vi "test1.vi"() -> ()   [LabVIEW 2020]
uses:
  <vilib>/DAQmx/write.llb/DAQmx Write (Digital Wfm 1Chan NSamp).vi
  <vilib>/DAQmx/create/channels.llb/DAQmx Create Channel (DO-Digital Output).vi
  <vilib>/Waveform/DWDTOps.llb/DWDT Digital to Boolean Array.vi
  <vilib>/DAQmx/configure/timing.llb/DAQmx Timing (Sample Clock).vi
  <vilib>/Waveform/DWDTOps.llb/DWDT Uncompress Digital.vi
  <vilib>/DAQmx/miscellaneous.llb/DAQmx Fill In Error Info.vi
  <resource>/objmgr/daqmx.rc
panel:
  out "number of samples written per channel":u32
  out "SampClk.Rate":dbl
  in  "stop":bool
  in  "Generate Stimuli":bool=TRUE
  in  "Sol Stim Parameters":cluster{"Fs":dbl, "Samples":dbl}
  in  "LED Stim Parameters":cluster{"Fs":dbl, "Samples":dbl}
  in  "Sol Duty Cycle (%)":dbl=10.0
  in  "Sol Freq":dbl=1.0
  in  "Sol Dur (s)":dbl=1.0
  in  "LED Duty Cycle (%)":dbl=10.0
  in  "LED Freq":dbl=10.0
  in  "LED Dur (s)":dbl=2.0
  out "Stimulus Order":digitalwaveform[](graph)=[{"t0"=timestamp(0 s since 1904-01-01), "dt"=5e-05, "Y"={"transitions"=[], "data"=array18000000x1[18000000 elements]}}, {"t0"=timestamp(0 s since 1904-01-01), "dt"=5e-05, "Y"={"transitions"=[], "data"=array18000000x1[18000000 elements]}}, {"t0"=timestamp(0 s since 1904-01-01), "dt"=5e-05, "Y"={"transitions"=[], "data"=array18000000x1[18000000 elements]}}, {"t0"=timestamp(0 s since 1904-01-01), "dt"=5e-05, "Y"={"transitions"=[], "data"=array18000000x1[18000000 elements]}}]
  out "Solenoid Stim":digitalwaveform(graph)={"t0"=timestamp(0 s since 1904-01-01), "dt"=5e-05, "Y"={"transitions"=[], "data"=array20000x1[20000 elements]}}
  in  "Trial Offset (s)":dbl=15.0
  in  "Interstim (s)":dbl=30.0
  in  "Right Pad":dbl=1.0
  in  "Left Pad":dbl=1.0
  in  "Auditory":dbl=1.0
  in  "LED":dbl
  in  "Time (min)":dbl(knob)=16.0 min=0.5 max=20.0 step=0.5 scale=0.0..20.0 scale format="%#_3g"
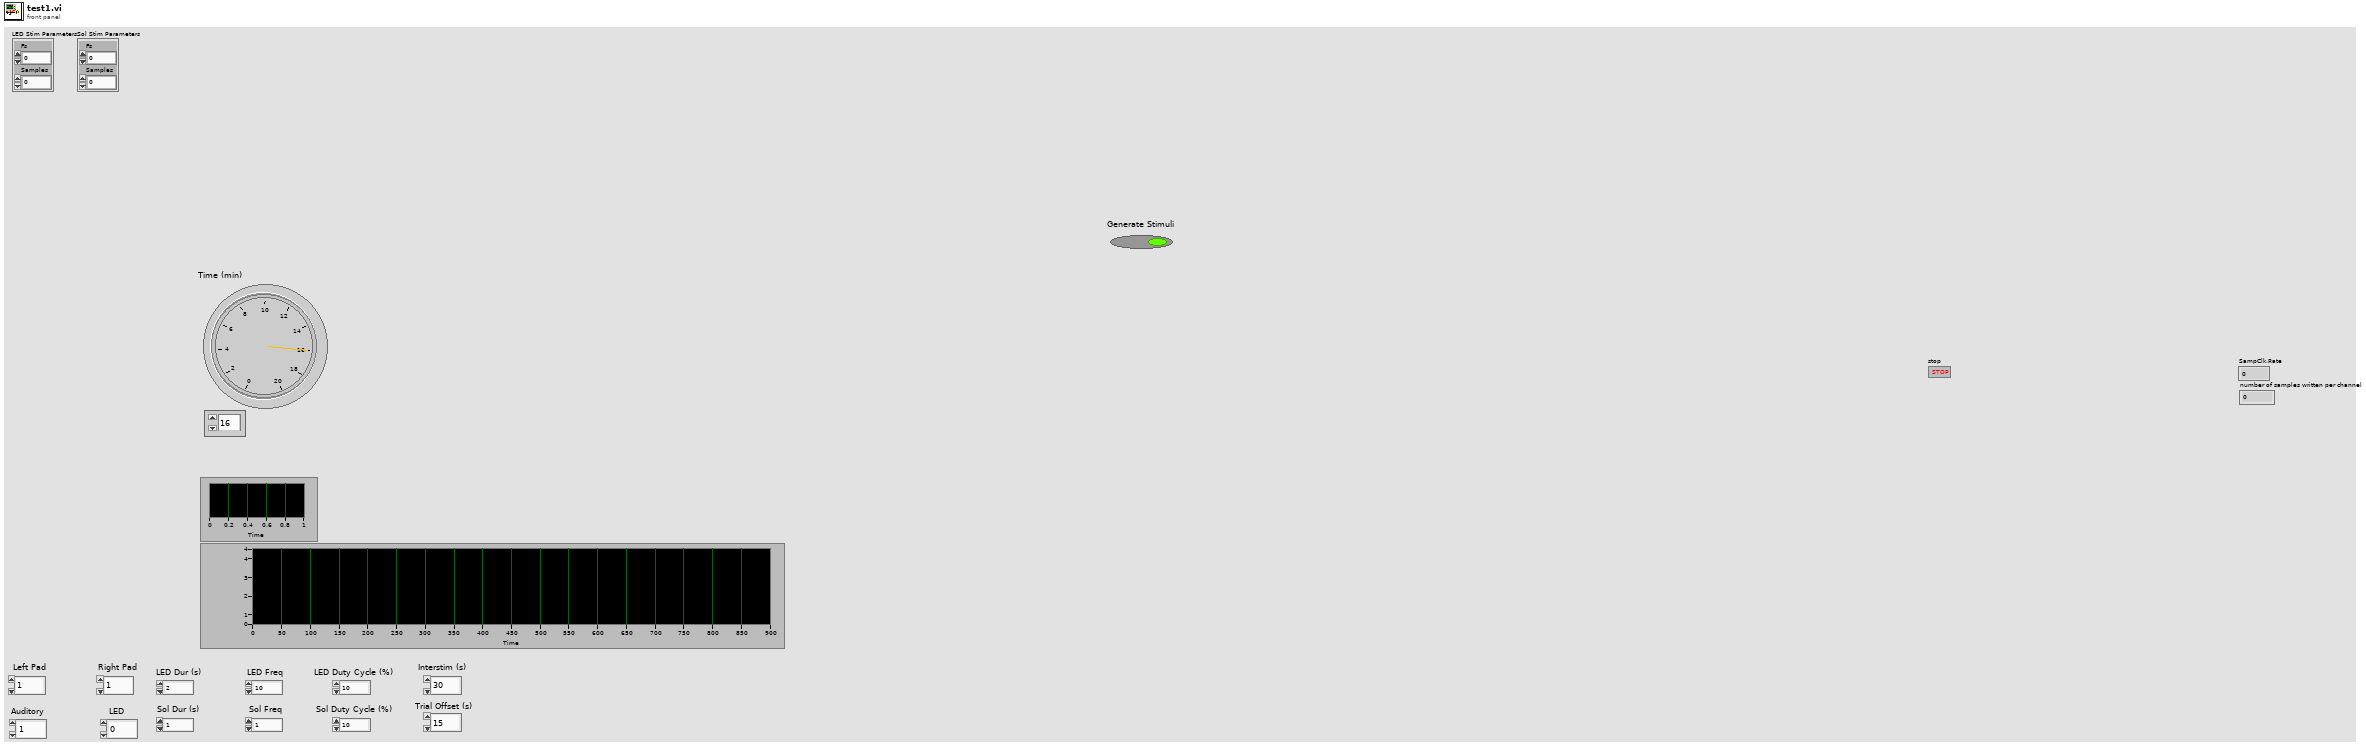
[diagram p1: front panel]
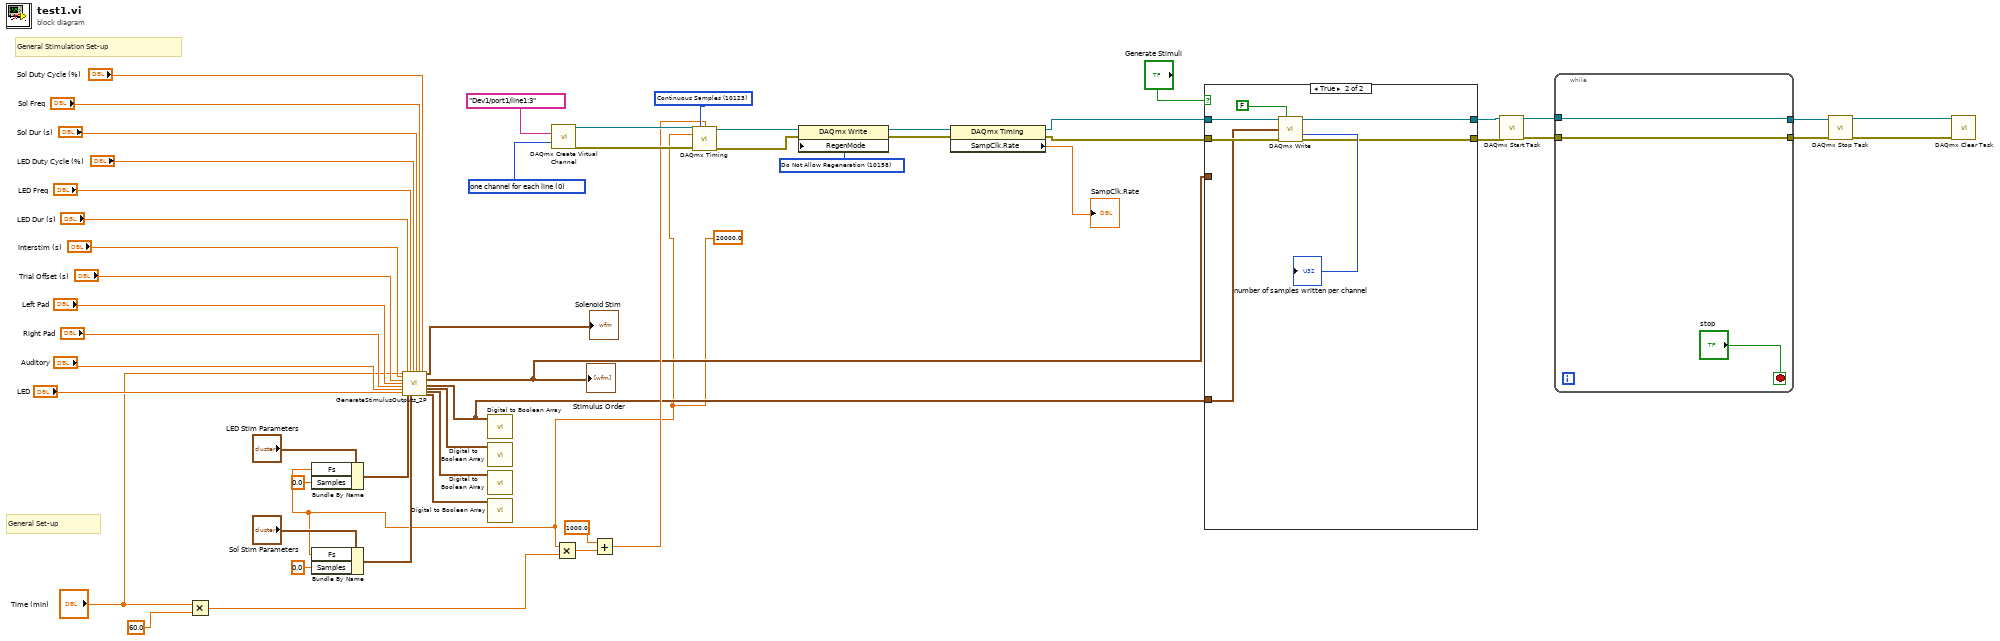
[diagram p0: block diagram]
diagram:
  w1 = 20000.0 ("rate")
  w34 = 10158 items=["Allow Regeneration"=10097, "Do Not Allow Regeneration"=10158] ("RegenMode")
  w35 = 10123 items=["Finite Samples"=10178, "Continuous Samples"=10123, "Hardware Timed Single Point"=12522] ("sample mode")
  w38 = 0 items=["one channel for each line", "one channel for all lines"] ("line grouping")
  # "General Stimulation Set-up"
  # "General Set-up"
  n1 = Multiply(x="Time (min)", y=60.0) -> (x*y=w19:dbl)
  n2 = Bundle By Name(cluster="LED Stim Parameters", "Fs"=w1, "Samples"=0.0) -> (w24:cluster{"Fs":dbl, "Samples":dbl})
  n3 = Bundle By Name(cluster="Sol Stim Parameters", "Fs"=w1, "Samples"=0.0) -> (w23:cluster{"Fs":dbl, "Samples":dbl})
  n4 = call "GenerateStimulusOutputs_2P.vi"("Trial duration (min)"="Time (min)", "Rest duration(s)"="Interstim (s)", "trial offset (s)"="Trial Offset (s)", "Left Pad"="Left Pad", "Right Pad"="Right Pad", "Auditory"="Auditory", "LED"="LED", "LED Stim Duration (s)"="LED Dur (s)", "LED Stim Parameters"=w24, "LED Frequency"="LED Freq", "Sol Stim Parameters"=w23, "LED duty cycle (%)"="LED Duty Cycle (%)", "Sol Stim Duration (s)"="Sol Dur (s)", "Sol Frequency"="Sol Freq", "Sol Duty Cycle (%)"="Sol Duty Cycle (%)") -> ("Solenoid Stim Waveforms"=→"Solenoid Stim":digitalwaveform, "Stimulus Digital Outputs"=w5:digitalwaveform[], "Left Pad Out"=w4:digitalwaveform, "Auditory Out"=w40:digitalwaveform, "Right Pad Out"=w39:digitalwaveform, "LED Out"=w18:digitalwaveform)  [unwired: 7 in]
  "Stimulus Order" <- w5
  n5 = call-poly <vilib>:"Digital to Boolean Array.vi"("digital waveform"=w4) -> ()  [unwired: 9 in, 2 out]
  n6 = call-poly <vilib>:"Digital to Boolean Array.vi"("digital waveform"=w40) -> ()  [unwired: 9 in, 2 out]
  n7 = call-poly <vilib>:"Digital to Boolean Array.vi"("digital waveform"=w39) -> ()  [unwired: 9 in, 2 out]
  n8 = call-poly <vilib>:"Digital to Boolean Array.vi"("digital waveform"=w18) -> ()  [unwired: 9 in, 2 out]
  n9 = call-poly <vilib>:"DAQmx Create Virtual Channel.vi"("lines"=tag "Dev1/port1/line1:3", "line grouping"=w38) -> ("task out"=w37:refnum<k21>, "error out"=w36:errorcluster)  [unwired: 12 in]
  n10 = Multiply(x=w1, y=w19) -> (x*y=w22:dbl)
  n11 = Add(x=1000.0, y=w22) -> (x+y=w20:dbl)
  n12 = call-poly <vilib>:"DAQmx Timing.vi"("task/channels in"=w37, "sample mode"=w35, "samples per channel"=w20, "rate"=w1, "error in"=w36) -> ("task out"=w31:refnum<k21>, "error out"=w30:errorcluster)  [unwired: 9 in]
  n13 = property class="DAQmx Write"(reference=w31, error in=w30, "RegenMode"=w34) -> (reference out=w32:refnum<k21>, error out=w33:errorcluster)
  n14 = property class="DAQmx Timing"(reference=w32, error in=w33) -> (reference out=w8:refnum<k21>, error out=w7:errorcluster, "SampClk.Rate"=→"SampClk.Rate":dbl)
  n15 = case shown="True" "Generate Stimuli" {
    tunnel: [w55 w62] -> w3
    tunnel: w8 -> [w55 w60]
    tunnel: w7 -> [w54 w59]
    tunnel: w5 -> [_ _]
    tunnel: w4 -> [_ w57]
    tunnel: [w54 w56] -> w2
    frame False {
    }
    frame True {
      n16 = call-poly <vilib>:"DAQmx Write.vi"("task/channels in"=w60, "auto start"=FALSE, "data"=w57, "error in"=w59) -> ("task out"=w62:refnum<k21>, "number of samples written per channel"=→"number of samples written per channel":u32, "error out"=w56:errorcluster)  [unwired: 9 in]
    }
  }
  n17 = call <vilib>:"DAQmx Start Task.vi"("task/channels in"=w3, "error in"=w2) -> ("task out"=w15:refnum<k21>, "error out"=w10:errorcluster)  [unwired: 12 in]
  n18 = while {
    tunnel: [w64] -> w14
    tunnel: w15 -> [w64]
    tunnel: w10 -> [w63]
    tunnel: [w63] -> w11
    stop <- "stop" stop-if-true
  }
  n19 = call <vilib>:"DAQmx Stop Task.vi"("task/channels in"=w14, "error in"=w11) -> ("task out"=w13:refnum<k21>, "error out"=w12:errorcluster)  [unwired: 12 in]
  n20 = call <vilib>:"DAQmx Clear Task.vi"("task in"=w13, "error in"=w12) -> ()  [unwired: 13 in, 1 out]
